vi "Set 664 Message Data.vi"(0 "MSG DATA In":u8[](array[numeric]), 5 "664 Parameter":T1, 7 "Value":dbl, 11 "error in (no error)":errorcluster) -> (4 "MSG DATA Out":u8[](array[numeric]) format="%x", 15 "error out":errorcluster)   [LabVIEW 2015, in "AIT 664 Custom Device.lvlib"]
doc: "Convert double to U8 array"
uses:
  AIT 664 Custom Device.lvlib
  Controls/664 -Param.ctl
panel:
  out "(hi.lo) 2":i16
  out "(hi.lo)":i32
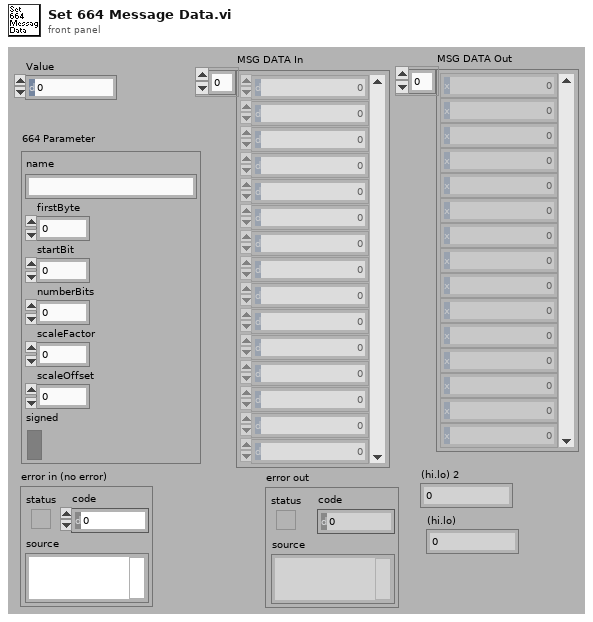
[diagram p1: front panel]
types:
  T1 = typedef "AIT 664 Custom Device.lvlib/664 -Param.ctl" = cluster{"name":string, "firstByte":i32, "startBit":i32, "numberBits":i32, "scaleFactor":dbl, "scaleOffset":dbl, "signed":bool}
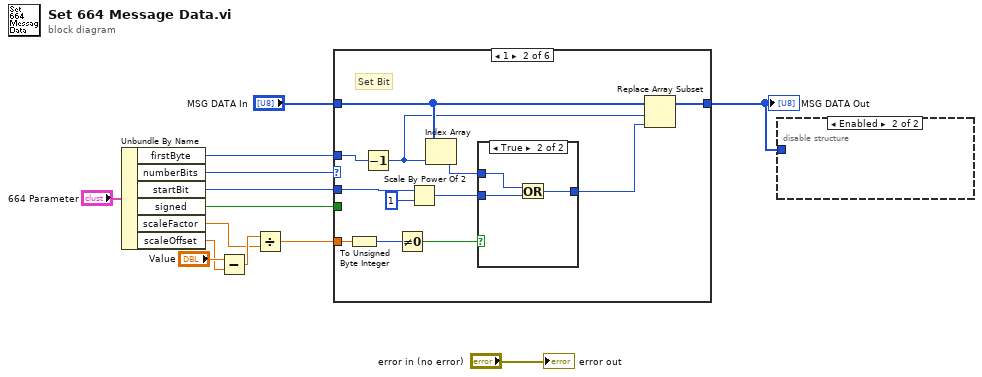
[diagram p0: block diagram]
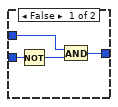
[diagram p3: hidden frame]
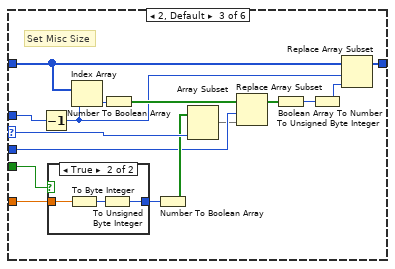
[diagram p4: hidden frame]
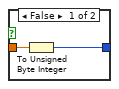
[diagram p5: hidden frame]
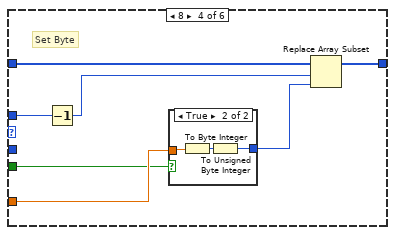
[diagram p6: hidden frame]
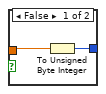
[diagram p7: hidden frame]
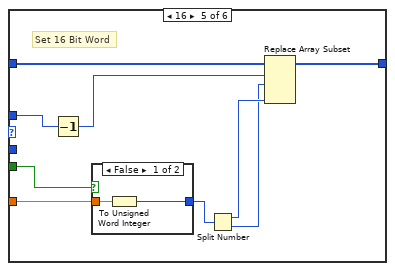
[diagram p8: hidden frame]
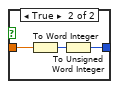
[diagram p9: hidden frame]
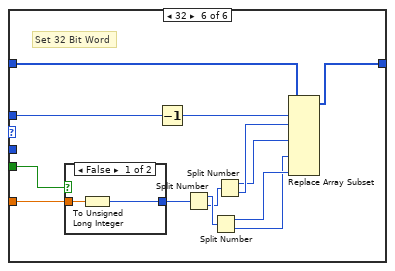
[diagram p10: hidden frame]
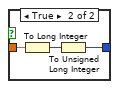
[diagram p11: hidden frame]
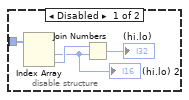
[diagram p12: hidden frame]
diagram:
  n1 = Unbundle By Name("664 Parameter") -> ("firstByte"=w11:i32, "numberBits"=w10:i32, "startBit"=w9:i32, "signed"=w8:bool, "scaleFactor"=w4:dbl, "scaleOffset"=w5:dbl)
  n2 = Subtract(x="Value", y=w5) -> (x-y=w7:dbl)
  n3 = Divide(x=w7, y=w4) -> (x/y=w3:dbl)
  n4 = case shown="1" w10 {
    selector: w10 -> [_ _ w45 _ _ _]
    tunnel: "MSG DATA In" -> [w14 w23 w37 w60 w74 w91]
    tunnel: w11 -> [_ w26 w46 w61 w75 w88]
    tunnel: w9 -> [_ w24 w41 _ _ _]
    tunnel: w8 -> [_ _ w48 w55 w71 w89]
    tunnel: w3 -> [_ w21 w49 w57 w72 w93]
    tunnel: [w14 w20 w35 w59 w70 w87] -> w1
    frame 0 {
      # "No Bits - Should not happen"
    }
    frame 1 {
      # "Set Bit"
      n5 = To Unsigned Byte Integer(number=w21) -> (unsigned 8bit integer=w19:u8)
      n6 = Decrement(x=w26) -> (x-1=w22:i32)
      n7 = Not Equal To 0?(x=w19) -> (x != 0?=w18:bool)
      n8 = Scale By Power Of 2(n=w24, x=u8 1) -> (x*2^n=w16:u8)
      n9 = Index Array(array=w23, index=w22) -> (element=w17:u8)
      n10 = case shown="True" w18 {
        tunnel: w17 -> [w28 w31]
        tunnel: w16 -> [w30 w33]
        tunnel: [w27 w32] -> w15
        frame False {
          n11 = Not(x=w30) -> (.not. x?=w29:u8)
          n12 = And(x=w28, y=w29) -> (x .and. y?=w27:u8)
        }
        frame True {
          n13 = Or(x=w31, y=w33) -> (x .or. y?=w32:u8)
        }
      }
      n14 = Replace Array Subset(array=w23, new element=w15, index=w22) -> (w20:u8[])
    }
    frame 2, Default {
      # "Set Misc Size"
      n15 = Decrement(x=w46) -> (x-1=w36:i32)
      n16 = case shown="True" w48 {
        tunnel: w49 -> [w51 w54]
        tunnel: [w50 w52] -> w44
        frame False {
          n17 = To Unsigned Byte Integer(number=w51) -> (unsigned 8bit integer=w50:u8)
        }
        frame True {
          n18 = To Byte Integer(number=w54) -> (8bit integer=w53:i8)
          n19 = To Unsigned Byte Integer(number=w53) -> (unsigned 8bit integer=w52:u8)
        }
      }
      n20 = Index Array(array=w37, index=w36) -> (element=w47:u8)
      n21 = Number To Boolean Array(number=w47) -> (Boolean array=w42:bool[])
      n22 = Number To Boolean Array(number=w44) -> (Boolean array=w43:bool[])
      n23 = Array Subset(array=w43, length=w45) -> (w40:bool[])  [unwired: 1 in]
      n24 = Replace Array Subset(array=w42, new element=w40, index=w41) -> (w38:bool[])
      n25 = Boolean Array To Number(Boolean array=w38) -> (number=w39:u32)
      n26 = To Unsigned Byte Integer(number=w39) -> (unsigned 8bit integer=w34:u8)
      n27 = Replace Array Subset(array=w37, new element=w34, index=w36) -> (w35:u8[])
    }
    frame 8 {
      # "Set Byte"
      n28 = Decrement(x=w61) -> (x-1=w58:i32)
      n29 = case shown="True" w55 {
        tunnel: w57 -> [w63 w64]
        tunnel: [w62 w66] -> w56
        frame False {
          n30 = To Unsigned Byte Integer(number=w63) -> (unsigned 8bit integer=w62:u8)
        }
        frame True {
          n31 = To Byte Integer(number=w64) -> (8bit integer=w65:i8)
          n32 = To Unsigned Byte Integer(number=w65) -> (unsigned 8bit integer=w66:u8)
        }
      }
      n33 = Replace Array Subset(array=w60, new element=w56, index=w58) -> (w59:u8[])
    }
    frame 16 {
      # "Set 16 Bit Word"
      n34 = Decrement(x=w75) -> (x-1=w73:i32)
      n35 = case shown="False" w71 {
        tunnel: w72 -> [w77 w80]
        tunnel: [w76 w78] -> w69
        frame False {
          n36 = To Unsigned Word Integer(number=w77) -> (unsigned 16bit integer=w76:u16)
        }
        frame True {
          n37 = To Word Integer(number=w80) -> (16bit integer=w79:i16)
          n38 = To Unsigned Word Integer(number=w79) -> (unsigned 16bit integer=w78:u16)
        }
      }
      n39 = Split Number(x=w69) -> (hi(x)=w68:u8, lo(x)=w67:u8)
      n40 = Replace Array Subset(array=w74, new element #1=w67, index #1=w73, new element #2=w68) -> (w70:u8[])  [unwired: 1 in]
    }
    frame 32 {
      # "Set 32 Bit Word"
      n41 = case shown="False" w89 {
        tunnel: w93 -> [w95 w98]
        tunnel: [w94 w96] -> w92
        frame False {
          n42 = To Unsigned Long Integer(number=w95) -> (unsigned 32bit integer=w94:u32)
        }
        frame True {
          n43 = To Long Integer(number=w98) -> (32bit integer=w97:i32)
          n44 = To Unsigned Long Integer(number=w97) -> (unsigned 32bit integer=w96:u32)
        }
      }
      n45 = Decrement(x=w88) -> (x-1=w90:i32)
      n46 = Split Number(x=w92) -> (hi(x)=w86:u16, lo(x)=w83:u16)
      n47 = Split Number(x=w86) -> (hi(x)=w85:u8, lo(x)=w84:u8)
      n48 = Split Number(x=w83) -> (hi(x)=w81:u8, lo(x)=w82:u8)
      n49 = Replace Array Subset(array=w91, new element #1=w82, index #1=w90, new element #2=w81, new element #3=w84, new element #4=w85) -> (w87:u8[])  [unwired: 3 in]
    }
  }
  "MSG DATA Out" <- w1
  n50 = disable-structure shown="Enabled" {
    disable-tunnel: w1 -> [w102 _]
    frame Disabled {
      n51 = Index Array(array=w102) -> (element #1=w99:u8, element #2=w101:u8)  [unwired: 2 in]
      "(hi.lo) 2" <- w99
      n52 = Join Numbers(hi=w101, lo=w99) -> ((hi.lo)=→"(hi.lo)":u16)
    }
    frame Enabled {
    }
  }
  "error out" <- "error in (no error)"
